vi "App - analyze RUS V6.vi"() -> ()   [LabVIEW 2015] (continued)
"z(0)"=-0.2711634458020681+0.39008831058364485i, "radius"=0.46500524213102634}}, "timestamp(min)"=628.25, "timestamp"=timestamp(3493765516 s since 1904-01-01), "Magn Field(T)"=0.0}, {"temperature"=96.968, "lorentzian"={"Amplitude"=0.00037146242302691187, "omega(0)"=668.0649075247303, "Gamma"=0.06217233966341157, "phase"=3.691468660230438, "Q"=10745.37183483038, "Norm  Ampl"=0.029107990080270388, "z (inf)"=0.2326634260645355-0.3951672463399738i, "4corners"={"z (-pi/2)"=-0.4111672463399738-0.2406634260645355i, "z(inf)"=0.2326634260645355-0.3951672463399738i, "z (pi/2)"=0.3871672463399738+0.2486634260645355i, "z center"=-0.01200000000000001+0.0040000000000000036i, "z(0)"=-0.2566634260645355+0.4031672463399738i, "radius"=0.4681823176971486}}, "timestamp(min)"=629.5666666701436, "timestamp"=timestamp(3493765595 s since 1904-01-01), "Magn Field(T)"=0.0}, {"temperature"=96.812, "lorentzian"={"Amplitude"=0.00038447207921998627, "omega(0)"=668.0660057593828, "Gamma"=0.06696620336364374, "phase"=3.806955565337118, "Q"=9976.166666215378, "Norm  Ampl"=0.030872979781580823, "z (inf)"=0.2726102759872714-0.350683705269581i, "4corners"={"z (-pi/2)"=-0.374683705269581-0.2726102759872714i, "z(inf)"=0.2726102759872714-0.350683705269581i, "z (pi/2)"=0.350683705269581+0.2966102759872714i, "z center"=-0.01200000000000001+0.01200000000000001i, "z(0)"=-0.2966102759872714+0.374683705269581i, "radius"=0.4610232957949339}}, "timestamp(min)"=630.8999999985099, "timestamp"=timestamp(3493765675 s since 1904-01-01), "Magn Field(T)"=0.0}, {"temperature"=96.655, "lorentzian"={"Amplitude"=0.000361199895859237, "omega(0)"=668.0603228410023, "Gamma"=0.0629920810816999, "phase"=3.775356755255857, "Q"=10605.465184973596, "Norm  Ampl"=0.029419314400986003, "z (inf)"=0.25656794858229404-0.372336300708436i, "4corners"={"z (-pi/2)"=-0.396336300708436-0.27256794858229405i, "z(inf)"=0.25656794858229404-0.372336300708436i, "z (pi/2)"=0.35633630070843597+0.28056794858229406i, "z center"=-0.020000000000000018+0.0040000000000000036i, "z(0)"=-0.29656794858229407+0.380336300708436i, "radius"=0.46703194902910955}}, "timestamp(min)"=632.2166666686535, "timestamp"=timestamp(3493765754 s since 1904-01-01), "Magn Field(T)"=0.0}, {"temperature"=96.507, "lorentzian"={"Amplitude"=0.00035745009367951465, "omega(0)"=668.0526848700105, "Gamma"=0.06285914936442166, "phase"=3.782468820239237, "Q"=10627.771639050034, "Norm  Ampl"=0.028980262367324632, "z (inf)"=0.2556518430633841-0.3655527717167506i, "4corners"={"z (-pi/2)"=-0.3895527717167506-0.27165184306338414i, "z(inf)"=0.2556518430633841-0.3655527717167506i, "z (pi/2)"=0.3495527717167506+0.27965184306338414i, "z center"=-0.020000000000000018+0.0040000000000000036i, "z(0)"=-0.29565184306338416+0.3735527717167506i, "radius"=0.4610349115498449}}, "timestamp(min)"=633.5500000044703, "timestamp"=timestamp(3493765834 s since 1904-01-01), "Magn Field(T)"=0.0}, {"temperature"=96.351, "lorentzian"={"Amplitude"=0.0003691797242721114, "omega(0)"=668.0459870419369, "Gamma"=0.06408388530782533, "phase"=3.8227658205621733, "Q"=10424.555000574557, "Norm  Ampl"=0.029587224824382054, "z (inf)"=0.2627317152722984-0.35466079325625405i, "4corners"={"z (-pi/2)"=-0.3866607932562541-0.2867317152722984i, "z(inf)"=0.2627317152722984-0.35466079325625405i, "z (pi/2)"=0.330660793256254+0.2947317152722984i, "z center"=-0.028000000000000025+0.0040000000000000036i, "z(0)"=-0.31873171527229843+0.36266079325625405i, "radius"=0.4616952402661069}}, "timestamp(min)"=634.8666666671634, "timestamp"=timestamp(3493765913 s since 1904-01-01), "Magn Field(T)"=0.0}, {"temperature"=96.204, "lorentzian"={"Amplitude"=0.00038180833108307917, "omega(0)"=668.0382438056512, "Gamma"=0.0652530874331081, "phase"=3.8620996852149454, "Q"=10237.649589997822, "Norm  Ampl"=0.02969485182794312, "z (inf)"=0.27224091953885815-0.33797353554027637i, "4corners"={"z (-pi/2)"=-0.3699735355402764-0.29624091953885817i, "z(inf)"=0.27224091953885815-0.33797353554027637i, "z (pi/2)"=0.31397353554027635+0.3042409195388582i, "z center"=-0.028000000000000025+0.0040000000000000036i, "z(0)"=-0.3282409195388582+0.3459735355402764i, "radius"=0.45507198197148524}}, "timestamp(min)"=636.183333337307, "timestamp"=timestamp(3493765992 s since 1904-01-01), "Magn Field(T)"=0.0}, {"temperature"=96.051, "lorentzian"={"Amplitude"=0.0003882934961133009, "omega(0)"=668.0317727144501, "Gamma"=0.06568797813583101, "phase"=3.9352495822111924, "Q"=10169.772181647602, "Norm  Ampl"=0.02993123400136465, "z (inf)"=0.2888486047387337-0.31552673906111356i, "4corners"={"z (-pi/2)"=-0.35552673906111354-0.32084860473873367i, "z(inf)"=0.2888486047387337-0.31552673906111356i, "z (pi/2)"=0.2835267390611136+0.3288486047387337i, "z center"=-0.035999999999999976+0.0040000000000000036i, "z(0)"=-0.36084860473873365+0.32352673906111357i, "radius"=0.4556577147110876}}, "timestamp(min)"=637.5166666656733, "timestamp"=timestamp(3493766072 s since 1904-01-01), "Magn Field(T)"=0.0}, {"temperature"=95.897, "lorentzian"={"Amplitude"=0.0003815839774204844, "omega(0)"=668.0229320244955, "Gamma"=0.06445033392425954, "phase"=3.977002601298967, "Q"=10364.925848321278, "Norm  Ampl"=0.029097485771713064, "z (inf)"=0.29079840497182946-0.2988803378584398i, "4corners"={"z (-pi/2)"=-0.3468803378584398-0.33079840497182944i, "z(inf)"=0.29079840497182946-0.2988803378584398i, "z (pi/2)"=0.25888033785843984+0.33879840497182945i, "z center"=-0.043999999999999984+0.0040000000000000036i, "z(0)"=-0.3787984049718294+0.3068803378584398i, "radius"=0.45147145096110314}}, "timestamp(min)"=638.8333333358169, "timestamp"=timestamp(3493766151 s since 1904-01-01), "Magn Field(T)"=0.0}, {"temperature"=95.75, "lorentzian"={"Amplitude"=0.0004135836601823012, "omega(0)"=668.0104558389754, "Gamma"=0.06731735153927441, "phase"=3.9838630372883417, "Q"=9923.302693351558, "Norm  Ampl"=0.030634815829311563, "z (inf)"=0.3035613371868464-0.29897918169328014i, "4corners"={"z (-pi/2)"=-0.3389791816932801-0.3355613371868464i, "z(inf)"=0.3035613371868464-0.29897918169328014i, "z (pi/2)"=0.26697918169328017+0.3435613371868464i, "z center"=-0.035999999999999976+0.0040000000000000036i, "z(0)"=-0.37556133718684637+0.30697918169328015i, "radius"=0.45508052721650133}}, "timestamp(min)"=640.1499999985099, "timestamp"=timestamp(3493766230 s since 1904-01-01), "Magn Field(T)"=0.0}, {"temperature"=95.599, "lorentzian"={"Amplitude"=0.00042216802189360146, "omega(0)"=668.0013835956787, "Gamma"=0.06780134474946373, "phase"=3.9776981169897643, "Q"=9852.332369867372, "Norm  Ampl"=0.0307062205288882, "z (inf)"=0.30005798229377045-0.30759507485352017i, "4corners"={"z (-pi/2)"=-0.33959507485352014-0.34005798229377043i, "z(inf)"=0.30005798229377045-0.30759507485352017i, "z (pi/2)"=0.2675950748535202+0.3320579822937704i, "z center"=-0.035999999999999976-0.0040000000000000036i, "z(0)"=-0.3720579822937704+0.29959507485352016i, "radius"=0.4528851255436357}}, "timestamp(min)"=641.4833333343267, "timestamp"=timestamp(3493766310 s since 1904-01-01), "Magn Field(T)"=0.0}, {"temperature"=95.455, "lorentzian"={"Amplitude"=0.0004523874054454233, "omega(0)"=667.9844280868045, "Gamma"=0.06782073622219846, "phase"=3.948222002818395, "Q"=9849.265361825519, "Norm  Ampl"=0.031118440336053946, "z (inf)"=0.3032591325695712-0.32148348753188644i, "4corners"={"z (-pi/2)"=-0.34548348753188646-0.33525913256957124i, "z(inf)"=0.3032591325695712-0.32148348753188644i, "z (pi/2)"=0.2894834875318864+0.32725913256957123i, "z center"=-0.028000000000000025-0.0040000000000000036i, "z(0)"=-0.35925913256957126+0.31348348753188643i, "radius"=0.45883371472261525}}, "timestamp(min)"=642.8000000044703, "timestamp"=timestamp(3493766389 s since 1904-01-01), "Magn Field(T)"=0.0}, {"temperature"=95.306, "lorentzian"={"Amplitude"=0.0004854419287925806, "omega(0)"=667.9730328624377, "Gamma"=0.07037414769947414, "phase"=3.891621301723143, "Q"=9491.738865740166, "Norm  Ampl"=0.032723058122378475, "z (inf)"=0.29696285365839886-0.3442166726157581i, "4corners"={"z (-pi/2)"=-0.3602166726157581-0.3209628536583989i, "z(inf)"=0.29696285365839886-0.3442166726157581i, "z (pi/2)"=0.3202166726157581+0.3129628536583989i, "z center"=-0.020000000000000018-0.0040000000000000036i, "z(0)"=-0.3369628536583989+0.3362166726157581i, "radius"=0.4649869190902186}}, "timestamp(min)"=644.1166666671634, "timestamp"=timestamp(3493766468 s since 1904-01-01), "Magn Field(T)"=0.0}, {"temperature"=95.156, "lorentzian"={"Amplitude"=0.0004910318217417332, "omega(0)"=667.9597690228534, "Gamma"=0.07026492453818647, "phase"=3.8418803163628708, "Q"=9506.304509867383, "Norm  Ampl"=0.03265446304858576, "z (inf)"=0.27949176570968204-0.3593616350093592i, "4corners"={"z (-pi/2)"=-0.3753616350093592-0.30349176570968206i, "z(inf)"=0.27949176570968204-0.3593616350093592i, "z (pi/2)"=0.33536163500935917+0.29549176570968205i, "z center"=-0.020000000000000018-0.0040000000000000036i, "z(0)"=-0.3194917657096821+0.3513616350093592i, "radius"=0.46473348207809184}}, "timestamp(min)"=645.4500000029802, "timestamp"=timestamp(3493766548 s since 1904-01-01), "Magn Field(T)"=0.0}, {"temperature"=95.012, "lorentzian"={"Amplitude"=0.0004787690427261217, "omega(0)"=667.9520044016398, "Gamma"=0.06706732978723035, "phase"=3.8089981908201227, "Q"=9959.424454808372, "Norm  Ampl"=0.031129732965038723, "z (inf)"=0.27528976862458415-0.36056246197020664i, "4corners"={"z (-pi/2)"=-0.37656246197020665-0.28328976862458416i, "z(inf)"=0.27528976862458415-0.36056246197020664i, "z (pi/2)"=0.35256246197020663+0.29128976862458417i, "z center"=-0.01200000000000001+0.0040000000000000036i, "z(0)"=-0.2992897686245842+0.36856246197020665i, "radius"=0.46415643896658965}}, "timestamp(min)"=646.7666666656733, "timestamp"=timestamp(3493766627 s since 1904-01-01), "Magn Field(T)"=0.0}, {"temperature"=94.866, "lorentzian"={"Amplitude"=0.0004761292193022266, "omega(0)"=667.9421204350114, "Gamma"=0.06630831442400692, "phase"=3.797924871572925, "Q"=10073.278535838983, "Norm  Ampl"=0.030739202330990468, "z (inf)"=0.270883513585858-0.363264549434754i, "4corners"={"z (-pi/2)"=-0.379264549434754-0.278883513585858i, "z(inf)"=0.270883513585858-0.363264549434754i, "z (pi/2)"=0.355264549434754+0.286883513585858i, "z center"=-0.01200000000000001+0.0040000000000000036i, "z(0)"=-0.294883513585858+0.371264549434754i, "radius"=0.4635799084626006}}, "timestamp(min)"=648.1000000014901, "timestamp"=timestamp(3493766707 s since 1904-01-01), "Magn Field(T)"=0.0}, {"temperature"=94.718, "lorentzian"={"Amplitude"=0.00047853053416581755, "omega(0)"=667.9314512587483, "Gamma"=0.06647786623615008, "phase"=3.7908834379562117, "Q"=10047.426144606505, "Norm  Ampl"=0.03076620958437617, "z (inf)"=0.2678212054341876-0.36462915903255366i, "4corners"={"z (-pi/2)"=-0.3806291590325537-0.2758212054341876i, "z(inf)"=0.2678212054341876-0.36462915903255366i, "z (pi/2)"=0.35662915903255366+0.2838212054341876i, "z center"=-0.01200000000000001+0.0040000000000000036i, "z(0)"=-0.2918212054341876+0.37262915903255367i, "radius"=0.46280380713612285}}, "timestamp(min)"=649.4166666641831, "timestamp"=timestamp(3493766786 s since 1904-01-01), "Magn Field(T)"=0.0}, {"temperature"=94.578, "lorentzian"={"Amplitude"=0.00047146401355324603, "omega(0)"=667.9245739426502, "Gamma"=0.06593817695384066, "phase"=3.8213286752443887, "Q"=10129.557788809114, "Norm  Ampl"=0.030202816047765486, "z (inf)"=0.2759230326145807-0.3522412452433142i, "4corners"={"z (-pi/2)"=-0.3682412452433142-0.2839230326145807i, "z(inf)"=0.2759230326145807-0.3522412452433142i, "z (pi/2)"=0.3442412452433142+0.2919230326145807i, "z center"=-0.01200000000000001+0.0040000000000000036i, "z(0)"=-0.2999230326145807+0.3602412452433142i, "radius"=0.45804748391677036}}, "timestamp(min)"=650.7333333343267, "timestamp"=timestamp(3493766865 s since 1904-01-01), "Magn Field(T)"=0.0}, {"temperature"=94.43, "lorentzian"={"Amplitude"=0.00047892263818113853, "omega(0)"=667.915672183135, "Gamma"=0.06684496153277945, "phase"=3.8401916398474936, "Q"=9992.012215544508, "Norm  Ampl"=0.0307040161855886, "z (inf)"=0.2834171775596786-0.3557305635687633i, "4corners"={"z (-pi/2)"=-0.3637305635687633-0.2994171775596786i, "z(inf)"=0.2834171775596786-0.3557305635687633i, "z (pi/2)"=0.3397305635687633+0.2914171775596786i, "z center"=-0.01200000000000001-0.0040000000000000036i, "z(0)"=-0.3074171775596786+0.3477305635687633i, "radius"=0.45933179526974455}}, "timestamp(min)"=652.0666666701436, "timestamp"=timestamp(3493766945 s since 1904-01-01), "Magn Field(T)"=0.0}, {"temperature"=94.292, "lorentzian"={"Amplitude"=0.0004657252078627852, "omega(0)"=667.9042185316268, "Gamma"=0.06477161400596823, "phase"=3.8153255665284904, "Q"=10311.680954408273, "Norm  Ampl"=0.029982133107207858, "z (inf)"=0.2768005918537779-0.3577476748367419i, "4corners"={"z (-pi/2)"=-0.3737476748367419-0.28480059185377793i, "z(inf)"=0.2768005918537779-0.3577476748367419i, "z (pi/2)"=0.3497476748367419+0.29280059185377794i, "z center"=-0.01200000000000001+0.0040000000000000036i, "z(0)"=-0.30080059185377794+0.3657476748367419i, "radius"=0.46289001080697517}}, "timestamp(min)"=653.3833333328366, "timestamp"=timestamp(3493767024 s since 1904-01-01), "Magn Field(T)"=0.0}, {"temperature"=94.146, "lorentzian"={"Amplitude"=0.00047004334807755914, "omega(0)"=667.8931568087993, "Gamma"=0.06620722920307591, "phase"=3.794159084218575, "Q"=10087.918870010191, "Norm  Ampl"=0.030640583697349073, "z (inf)"=0.26902377025013874-0.3637060990321072i, "4corners"={"z (-pi/2)"=-0.3797060990321072-0.27702377025013875i, "z(inf)"=0.26902377025013874-0.3637060990321072i, "z (pi/2)"=0.3557060990321072+0.28502377025013875i, "z center"=-0.01200000000000001+0.0040000000000000036i, "z(0)"=-0.29302377025013876+0.3717060990321072i, "radius"=0.4627981576357155}}, "timestamp(min)"=654.7000000029802, "timestamp"=timestamp(3493767103 s since 1904-01-01), "Magn Field(T)"=0.0}, {"temperature"=94.003, "lorentzian"={"Amplitude"=0.00047665410550718444, "omega(0)"=667.8785430669695, "Gamma"=0.06600452228276824, "phase"=3.7493809753851632, "Q"=10118.678538505721, "Norm  Ampl"=0.030401685578484956, "z (inf)"=0.25102715548226634-0.3741125652184201i, "4corners"={"z (-pi/2)"=-0.39011256521842014-0.25902715548226635i, "z(inf)"=0.25102715548226634-0.3741125652184201i, "z (pi/2)"=0.3661125652184201+0.26702715548226635i, "z center"=-0.01200000000000001+0.0040000000000000036i, "z(0)"=-0.27502715548226636+0.38211256521842013i, "radius"=0.4606000396191324}}, "timestamp(min)"=656.0333333313465, "timestamp"=timestamp(3493767183 s since 1904-01-01), "Magn Field(T)"=0.0}, {"temperature"=93.867, "lorentzian"={"Amplitude"=0.00048650304629364036, "omega(0)"=667.867203293899, "Gamma"=0.06682589428323253, "phase"=3.7348237629828676, "Q"=9994.137908027598, "Norm  Ampl"=0.03108362649647347, "z (inf)"=0.24803517339436904-0.38166842033020015i, "4corners"={"z (-pi/2)"=-0.39766842033020017-0.25603517339436904i, "z(inf)"=0.24803517339436904-0.38166842033020015i, "z (pi/2)"=0.37366842033020015+0.26403517339436905i, "z center"=-0.01200000000000001+0.0040000000000000036i, "z(0)"=-0.27203517339436906+0.38966842033020016i, "radius"=0.46514344222210796}}, "timestamp(min)"=657.3500000014901, "timestamp"=timestamp(3493767262 s since 1904-01-01), "Magn Field(T)"=0.0}, {"temperature"=93.722, "lorentzian"={"Amplitude"=0.0004956688777062957, "omega(0)"=667.8547807071961, "Gamma"=0.0674977463368087, "phase"=3.7437605166589782, "Q"=9894.47525217584, "Norm  Ampl"=0.03128536274271491, "z (inf)"=0.2505417919292505-0.3859767244686182i, "4corners"={"z (-pi/2)"=-0.3939767244686182-0.26654179192925054i, "z(inf)"=0.2505417919292505-0.3859767244686182i, "z (pi/2)"=0.3699767244686182+0.25854179192925053i, "z center"=-0.01200000000000001-0.0040000000000000036i, "z(0)"=-0.27454179192925054+0.3779767244686182i, "radius"=0.46350233067935753}}, "timestamp(min)"=658.683333337307, "timestamp"=timestamp(3493767342 s since 1904-01-01), "Magn Field(T)"=0.0}, {"temperature"=93.585, "lorentzian"={"Amplitude"=0.000482384363144179, "omega(0)"=667.8418460648647, "Gamma"=0.06604388460816402, "phase"=3.731195401069006, "Q"=10112.092134300492, "Norm  Ampl"=0.030626323452688318, "z (inf)"=0.24584645857021942-0.38143197531309236i, "4corners"={"z (-pi/2)"=-0.3974319753130924-0.2538464585702194i, "z(inf)"=0.24584645857021942-0.38143197531309236i, "z (pi/2)"=0.37343197531309236+0.26184645857021943i, "z center"=-0.01200000000000001+0.0040000000000000036i, "z(0)"=-0.26984645857021944+0.38943197531309237i, "radius"=0.4637268633484113}}, "timestamp(min)"=660.0, "timestamp"=timestamp(3493767421 s since 1904-01-01), "Magn Field(T)"=0.0}, {"temperature"=93.444, "lorentzian"={"Amplitude"=0.00048781220349119976, "omega(0)"=667.8284078259741, "Gamma"=0.06779248490994184, "phase"=3.7207259148041842, "Q"=9851.068429091265, "Norm  Ampl"=0.031501770847735304, "z (inf)"=0.24231844551293596-0.38490753149851276i, "4corners"={"z (-pi/2)"=-0.40090753149851277-0.25031844551293597i, "z(inf)"=0.24231844551293596-0.38490753149851276i, "z (pi/2)"=0.37690753149851275+0.258318445512936i, "z center"=-0.01200000000000001+0.0040000000000000036i, "z(0)"=-0.266318445512936+0.39290753149851276i, "radius"=0.46467939461997115}}, "timestamp(min)"=661.3166666701436, "timestamp"=timestamp(3493767500 s since 1904-01-01), "Magn Field(T)"=0.0}, {"temperature"=93.303, "lorentzian"={"Amplitude"=0.0004977863242643817, "omega(0)"=667.8174456972619, "Gamma"=0.06925915720810301, "phase"=3.733369961748711, "Q"=9642.298182905555, "Norm  Ampl"=0.03210673818426036, "z (inf)"=0.2465986694380145-0.3887434164619287i, "4corners"={"z (-pi/2)"=-0.39674341646192873-0.2625986694380145i, "z(inf)"=0.2465986694380145-0.3887434164619287i, "z (pi/2)"=0.3727434164619287+0.2545986694380145i, "z center"=-0.01200000000000001-0.0040000000000000036i, "z(0)"=-0.2705986694380145+0.3807434164619287i, "radius"=0.463573908180679}}, "timestamp(min)"=662.6499999985099, "timestamp"=timestamp(3493767580 s since 1904-01-01), "Magn Field(T)"=0.0}, {"temperature"=93.168, "lorentzian"={"Amplitude"=0.00048225409501391443, "omega(0)"=667.8098934060879, "Gamma"=0.06771518067251926, "phase"=3.7456795533249925, "Q"=9862.04107814046, "Norm  Ampl"=0.031358841542932885, "z (inf)"=0.2510453154387986-0.3771403549090192i, "4corners"={"z (-pi/2)"=-0.3931403549090192-0.2590453154387986i, "z(inf)"=0.2510453154387986-0.3771403549090192i, "z (pi/2)"=0.3691403549090192+0.2670453154387986i, "z center"=-0.01200000000000001+0.0040000000000000036i, "z(0)"=-0.2750453154387986+0.3851403549090192i, "radius"=0.46309913421908944}}, "timestamp(min)"=663.9666666686535, "timestamp"=timestamp(3493767659 s since 1904-01-01), "Magn Field(T)"=0.0}, {"temperature"=93.028, "lorentzian"={"Amplitude"=0.0004824745179479892, "omega(0)"=667.7999931838958, "Gamma"=0.06758256658053667, "phase"=3.763405165125436, "Q"=9881.246406765169, "Norm  Ampl"=0.031281978812503275, "z (inf)"=0.25762642400328667-0.38023227467776743i, "4corners"={"z (-pi/2)"=-0.38823227467776744-0.2736264240032867i, "z(inf)"=0.25762642400328667-0.38023227467776743i, "z (pi/2)"=0.3642322746777674+0.2656264240032867i, "z center"=-0.01200000000000001-0.0040000000000000036i, "z(0)"=-0.2816264240032867+0.3722322746777674i, "radius"=0.4628705359277119}}, "timestamp(min)"=665.2833333313465, "timestamp"=timestamp(3493767738 s since 1904-01-01), "Magn Field(T)"=0.0}, {"temperature"=92.895, "lorentzian"={"Amplitude"=0.00046952632702334146, "omega(0)"=667.7879029943412, "Gamma"=0.0659901281238434, "phase"=3.723190998312637, "Q"=10119.512144924258, "Norm  Ampl"=0.030488656955698742, "z (inf)"=0.24181454637365946-0.3820559902589959i, "4corners"={"z (-pi/2)"=-0.3980559902589959-0.24981454637365946i, "z(inf)"=0.24181454637365946-0.3820559902589959i, "z (pi/2)"=0.3740559902589959+0.25781454637365947i, "z center"=-0.01200000000000001+0.0040000000000000036i, "z(0)"=-0.2658145463736595+0.3900559902589959i, "radius"=0.46201845370690603}}, "timestamp(min)"=666.6166666671634, "timestamp"=timestamp(3493767818 s since 1904-01-01), "Magn Field(T)"=0.0}, {"temperature"=92.755, "lorentzian"={"Amplitude"=0.0004533781628719222, "omega(0)"=667.7767811952523, "Gamma"=0.06357707675527592, "phase"=3.7161636244174314, "Q"=10503.420655304619, "Norm  Ampl"=0.029386934028224773, "z (inf)"=0.23120776305430374-0.38400373351334605i, "4corners"={"z (-pi/2)"=-0.40800373351334607-0.24720776305430375i, "z(inf)"=0.23120776305430374-0.38400373351334605i, "z (pi/2)"=0.36800373351334603+0.25520776305430376i, "z center"=-0.020000000000000018+0.0040000000000000036i, "z(0)"=-0.2712077630543038+0.39200373351334605i, "radius"=0.4622253102536066}}, "timestamp(min)"=667.933333337307, "timestamp"=timestamp(3493767897 s since 1904-01-01), "Magn Field(T)"=0.0}, {"temperature"=92.618, "lorentzian"={"Amplitude"=0.0004725360269472116, "omega(0)"=667.766686685923, "Gamma"=0.06603299924648035, "phase"=3.718541594649695, "Q"=10112.620876016259, "Norm  Ampl"=0.03057472850998967, "z (inf)"=0.2405642593646345-0.384072966292819i, "4corners"={"z (-pi/2)"=-0.400072966292819-0.2485642593646345i, "z(inf)"=0.2405642593646345-0.384072966292819i, "z (pi/2)"=0.376072966292819+0.2565642593646345i, "z center"=-0.01200000000000001+0.0040000000000000036i, "z(0)"=-0.2645642593646345+0.392072966292819i, "radius"=0.4630219565805857}}, "timestamp(min)"=669.2666666656733, "timestamp"=timestamp(3493767977 s since 1904-01-01), "Magn Field(T)"=0.0}, {"temperature"=92.485, "lorentzian"={"Amplitude"=0.0004628266939696805, "omega(0)"=667.7537699797824, "Gamma"=0.06509770931054754, "phase"=3.7185205526120066, "Q"=10257.71531828062, "Norm  Ampl"=0.030151235786846406, "z (inf)"=0.2326362554983411-0.3842014578439372i, "4corners"={"z (-pi/2)"=-0.40820145784393724-0.24863625549834112i, "z(inf)"=0.2326362554983411-0.3842014578439372i, "z (pi/2)"=0.3682014578439372+0.2566362554983411i, "z center"=-0.020000000000000018+0.0040000000000000036i, "z(0)"=-0.27263625549834114+0.39220145784393723i, "radius"=0.4631689210907628}}, "timestamp(min)"=670.5833333358169, "timestamp"=timestamp(3493768056 s since 1904-01-01), "Magn Field(T)"=0.0}, {"temperature"=92.348, "lorentzian"={"Amplitude"=0.0004709340282676857, "omega(0)"=667.7441411520185, "Gamma"=0.06634297124541383, "phase"=3.7335153124062965, "Q"=10065.032189799285, "Norm  Ampl"=0.030723334211136075, "z (inf)"=0.23838936327255184-0.3803113449909337i, "4corners"={"z (-pi/2)"=-0.40431134499093374-0.25438936327255185i, "z(inf)"=0.23838936327255184-0.3803113449909337i, "z (pi/2)"=0.3643113449909337+0.26238936327255186i, "z center"=-0.020000000000000018+0.0040000000000000036i, "z(0)"=-0.27838936327255187+0.3883113449909337i, "radius"=0.46309855640148057}}, "timestamp(min)"=671.8999999985099, "timestamp"=timestamp(3493768135 s since 1904-01-01), "Magn Field(T)"=0.0}, {"temperature"=92.218, "lorentzian"={"Amplitude"=0.0004646839205690204, "omega(0)"=667.7346507175026, "Gamma"=0.0656240651590833, "phase"=3.75255081841295, "Q"=10175.149148392535, "Norm  Ampl"=0.030385059677175152, "z (inf)"=0.24561090162017518-0.3752566651128105i, "4corners"={"z (-pi/2)"=-0.3992566651128105-0.2616109016201752i, "z(inf)"=0.24561090162017518-0.3752566651128105i, "z (pi/2)"=0.35925666511281046+0.2696109016201752i, "z center"=-0.020000000000000018+0.0040000000000000036i, "z(0)"=-0.2856109016201752+0.3832566651128105i, "radius"=0.46301702894383145}}, "timestamp(min)"=673.2333333343267, "timestamp"=timestamp(3493768215 s since 1904-01-01), "Magn Field(T)"=0.0}, {"temperature"=92.082, "lorentzian"={"Amplitude"=0.0004749862394250107, "omega(0)"=667.7218411788447, "Gamma"=0.06705767219373826, "phase"=3.7603842163008987, "Q"=9957.426485812244, "Norm  Ampl"=0.03103865948557628, "z (inf)"=0.24848549273528175-0.37304069686884916i, "4corners"={"z (-pi/2)"=-0.3970406968688492-0.26448549273528177i, "z(inf)"=0.24848549273528175-0.37304069686884916i, "z (pi/2)"=0.35704069686884915+0.2724854927352818i, "z center"=-0.020000000000000018+0.0040000000000000036i, "z(0)"=-0.2884854927352818+0.38104069686884917i, "radius"=0.4628651498057014}}, "timestamp(min)"=674.5500000044703, "timestamp"=timestamp(3493768294 s since 1904-01-01), "Magn Field(T)"=0.0}, {"temperature"=91.948, "lorentzian"={"Amplitude"=0.00048240630679528417, "omega(0)"=667.7090832290504, "Gamma"=0.06807373016118351, "phase"=3.761077209038164, "Q"=9808.61606449453, "Norm  Ampl"=0.031227719593183583, "z (inf)"=0.23834797737965352-0.36949087855823637i, "4corners"={"z (-pi/2)"=-0.4014908785582364-0.26234797737965354i, "z(inf)"=0.23834797737965352-0.36949087855823637i, "z (pi/2)"=0.34549087855823635+0.27034797737965355i, "z center"=-0.028000000000000025+0.0040000000000000036i, "z(0)"=-0.29434797737965357+0.3774908785582364i, "radius"=0.4587337805529866}}, "timestamp(min)"=675.8666666671634, "timestamp"=timestamp(3493768373 s since 1904-01-01), "Magn Field(T)"=0.0}, {"temperature"=91.818, "lorentzian"={"Amplitude"=0.00046187913692467586, "omega(0)"=667.6987650095127, "Gamma"=0.06501069688502076, "phase"=3.7818049219720504, "Q"=10270.598486129418, "Norm  Ampl"=0.029800728728416378, "z (inf)"=0.24583082565039227-0.3636204223463083i, "4corners"={"z (-pi/2)"=-0.39562042234630834-0.2698308256503923i, "z(inf)"=0.24583082565039227-0.3636204223463083i, "z (pi/2)"=0.3396204223463083+0.2778308256503923i, "z center"=-0.028000000000000025+0.0040000000000000036i, "z(0)"=-0.3018308256503923+0.3716204223463083i, "radius"=0.45839731238572246}}, "timestamp(min)"=677.2000000029802, "timestamp"=timestamp(3493768453 s since 1904-01-01), "Magn Field(T)"=0.0}, {"temperature"=91.685, "lorentzian"={"Amplitude"=0.00048772981058133426, "omega(0)"=667.6847550615028, "Gamma"=0.06909515397897131, "phase"=3.8213110627573736, "Q"=9663.264593993214, "Norm  Ampl"=0.03163038100550472, "z (inf)"=0.25174863771982026-0.35203829662944414i, "4corners"={"z (-pi/2)"=-0.3920382966294441-0.28374863771982023i, "z(inf)"=0.25174863771982026-0.35203829662944414i, "z (pi/2)"=0.32003829662944416+0.29174863771982024i, "z center"=-0.035999999999999976+0.0040000000000000036i, "z(0)"=-0.3237486377198202+0.36003829662944414i, "radius"=0.45778002050811306}}, "timestamp(min)"=678.5166666656733, "timestamp"=timestamp(3493768532 s since 1904-01-01), "Magn Field(T)"=0.0}, {"temperature"=91.557, "lorentzian"={"Amplitude"=0.0004936970308438804, "omega(0)"=667.6716677581467, "Gamma"=0.06917469758289295, "phase"=3.7984123962847027, "Q"=9651.96366717855, "Norm  Ampl"=0.03174648182411007, "z (inf)"=0.2522245068977959-0.35944573170689686i, "4corners"={"z (-pi/2)"=-0.3914457317068969-0.27622450689779593i, "z(inf)"=0.2522245068977959-0.35944573170689686i, "z (pi/2)"=0.33544573170689684+0.28422450689779594i, "z center"=-0.028000000000000025+0.0040000000000000036i, "z(0)"=-0.30822450689779596+0.36744573170689687i, "radius"=0.45893199295982245}}, "timestamp(min)"=679.8500000014901, "timestamp"=timestamp(3493768612 s since 1904-01-01), "Magn Field(T)"=0.0}, {"temperature"=91.423, "lorentzian"={"Amplitude"=0.0005094399076372343, "omega(0)"=667.6622092104991, "Gamma"=0.07106029145812462, "phase"=3.881324924167042, "Q"=9395.71447724709, "Norm  Ampl"=0.03277559689637478, "z (inf)"=0.2829149636577557-0.3366918731694022i, "4corners"={"z (-pi/2)"=-0.3686918731694022-0.3069149636577557i, "z(inf)"=0.2829149636577557-0.3366918731694022i, "z (pi/2)"=0.31269187316940217+0.31491496365775573i, "z center"=-0.028000000000000025+0.0040000000000000036i, "z(0)"=-0.33891496365775575+0.3446918731694022i, "radius"=0.4612364546195147}}, "timestamp(min)"=681.1666666641831, "timestamp"=timestamp(3493768691 s since 1904-01-01), "Magn Field(T)"=0.0}, {"temperature"=91.291, "lorentzian"={"Amplitude"=0.0005088040446388636, "omega(0)"=667.6494194591486, "Gamma"=0.07122298109703128, "phase"=3.860166057202675, "Q"=9374.072935104616, "Norm  Ampl"=0.03258903067532576, "z (inf)"=0.27321925003049036-0.34042886777923675i, "4corners"={"z (-pi/2)"=-0.3724288677792368-0.2972192500304904i, "z(inf)"=0.27321925003049036-0.34042886777923675i, "z (pi/2)"=0.31642886777923673+0.3052192500304904i, "z center"=-0.028000000000000025+0.0040000000000000036i, "z(0)"=-0.3292192500304904+0.34842886777923676i, "radius"=0.4575634180620409}}, "timestamp(min)"=682.4833333343267, "timestamp"=timestamp(3493768770 s since 1904-01-01), "Magn Field(T)"=0.0}, {"temperature"=91.167, "lorentzian"={"Amplitude"=0.000510744332757808, "omega(0)"=667.6370796373111, "Gamma"=0.0716029354059644, "phase"=3.865224682997533, "Q"=9324.157953190535, "Norm  Ampl"=0.03278392731323275, "z (inf)"=0.27515231362484527-0.34712095541253063i, "4corners"={"z (-pi/2)"=-0.37112095541253065-0.3071523136248453i, "z(inf)"=0.27515231362484527-0.34712095541253063i, "z (pi/2)"=0.3151209554125306+0.2991523136248453i, "z center"=-0.028000000000000025-0.0040000000000000036i, "z(0)"=-0.3311523136248453+0.3391209554125306i, "radius"=0.45785730888487997}}, "timestamp(min)"=683.8166666701436, "timestamp"=timestamp(3493768850 s since 1904-01-01), "Magn Field(T)"=0.0}, {"temperature"=91.035, "lorentzian"={"Amplitude"=0.0005141802984750622, "omega(0)"=667.6271523663532, "Gamma"=0.0719675199748464, "phase"=3.826833710973994, "Q"=9276.784202091412, "Norm  Ampl"=0.032806058987522896, "z (inf)"=0.2524861359147123-0.3489457864081325i, "4corners"={"z (-pi/2)"=-0.3889457864081325-0.2844861359147123i, "z(inf)"=0.2524861359147123-0.3489457864081325i, "z (pi/2)"=0.31694578640813253+0.2924861359147123i, "z center"=-0.035999999999999976+0.0040000000000000036i, "z(0)"=-0.32448613591471226+0.3569457864081325i, "radius"=0.45584534521946907}}, "timestamp(min)"=685.1333333328366, "timestamp"=timestamp(3493768929 s since 1904-01-01), "Magn Field(T)"=0.0}, {"temperature"=90.91, "lorentzian"={"Amplitude"=0.0005028221303766884, "omega(0)"=667.616063077065, "Gamma"=0.07025360423713384, "phase"=3.8495426280010117, "Q"=9502.943946101263, "Norm  Ampl"=0.03210925964867006, "z (inf)"=0.26120805162066535-0.34321768770733674i, "4corners"={"z (-pi/2)"=-0.3832176877073367-0.2932080516206653i, "z(inf)"=0.26120805162066535-0.34321768770733674i, "z (pi/2)"=0.31121768770733677+0.30120805162066533i, "z center"=-0.035999999999999976+0.0040000000000000036i, "z(0)"=-0.3332080516206653+0.35121768770733675i, "radius"=0.45704786248814433}}, "timestamp(min)"=686.4500000029802, "timestamp"=timestamp(3493769008 s since 1904-01-01), "Magn Field(T)"=0.0}, {"temperature"=90.778, "lorentzian"={"Amplitude"=0.000496497929184537, "omega(0)"=667.5996159742031, "Gamma"=0.06890055492897058, "phase"=3.859639780398612, "Q"=9689.32132204784, "Norm  Ampl"=0.03137956944971089, "z (inf)"=0.26363614673359875-0.33898275837264435i, "4corners"={"z (-pi/2)"=-0.37898275837264433-0.2956361467335987i, "z(inf)"=0.26363614673359875-0.33898275837264435i, "z (pi/2)"=0.3069827583726444+0.30363614673359873i, "z center"=-0.035999999999999976+0.0040000000000000036i, "z(0)"=-0.3356361467335987+0.34698275837264436i, "radius"=0.4554327535106214}}, "timestamp(min)"=687.7833333313465, "timestamp"=timestamp(3493769088 s since 1904-01-01), "Magn Field(T)"=0.0}, {"temperature"=90.65, "lorentzian"={"Amplitude"=0.000499948600021398, "omega(0)"=667.5849862740106, "Gamma"=0.06954975580707387, "phase"=3.849891148655935, "Q"=9598.667580168712, "Norm  Ampl"=0.03138623678832294, "z (inf)"=0.25757515087784166-0.3387316327279606i, "4corners"={"z (-pi/2)"=-0.37873163272796057-0.28957515087784164i, "z(inf)"=0.25757515087784166-0.3387316327279606i, "z (pi/2)"=0.3067316327279606+0.29757515087784164i, "z center"=-0.035999999999999976+0.0040000000000000036i, "z(0)"=-0.3295751508778416+0.3467316327279606i, "radius"=0.4512774548826045}}, "timestamp(min)"=689.1000000014901, "timestamp"=timestamp(3493769167 s since 1904-01-01), "Magn Field(T)"=0.0}, {"temperature"=90.526, "lorentzian"={"Amplitude"=0.0005221121875696492, "omega(0)"=667.5706432660058, "Gamma"=0.0719106912079188, "phase"=3.8795533190442146, "Q"=9283.329530734547, "Norm  Ampl"=0.03259818591965365, "z (inf)"=0.2689814193704261-0.33138143772648987i, "4corners"={"z (-pi/2)"=-0.37138143772648985-0.30098141937042605i, "z(inf)"=0.2689814193704261-0.33138143772648987i, "z (pi/2)"=0.2993814377264899+0.30898141937042606i, "z center"=-0.035999999999999976+0.0040000000000000036i, "z(0)"=-0.34098141937042603+0.3393814377264899i, "radius"=0.4533148739371862}}, "timestamp(min)"=690.4166666641831, "timestamp"=timestamp(3493769246 s since 1904-01-01), "Magn Field(T)"=0.0}, {"temperature"=90.397, "lorentzian"={"Amplitude"=0.0005333126804893269, "omega(0)"=667.555832927336, "Gamma"=0.07307015936595498, "phase"=3.867011857823234, "Q"=9135.82013122535, "Norm  Ampl"=0.03301691741317805, "z (inf)"=0.2637810086163199-0.3340855235035937i, "4corners"={"z (-pi/2)"=-0.3740855235035937-0.2957810086163199i, "z(inf)"=0.2637810086163199-0.3340855235035937i, "z (pi/2)"=0.30208552350359374+0.3037810086163199i, "z center"=-0.035999999999999976+0.0040000000000000036i, "z(0)"=-0.3357810086163199+0.3420855235035937i, "radius"=0.4518522704709107}}, "timestamp(min)"=691.75, "timestamp"=timestamp(3493769326 s since 1904-01-01), "Magn Field(T)"=0.0}, {"temperature"=90.276, "lorentzian"={"Amplitude"=0.0005418855418945078, "omega(0)"=667.5428492141318, "Gamma"=0.07467380998758522, "phase"=3.887607241567496, "Q"=8939.450783683238, "Norm  Ampl"=0.03363448014434847, "z (inf)"=0.2697069491564103-0.32678733838832924i, "4corners"={"z (-pi/2)"=-0.3667873383883292-0.3017069491564103i, "z(inf)"=0.2697069491564103-0.32678733838832924i, "z (pi/2)"=0.29478733838832927+0.3097069491564103i, "z center"=-0.035999999999999976+0.0040000000000000036i, "z(0)"=-0.34170694915641026+0.33478733838832925i, "radius"=0.45041869632660125}}, "timestamp(min)"=693.0666666701436, "timestamp"=timestamp(3493769405 s since 1904-01-01), "Magn Field(T)"=0.0}, {"temperature"=90.146, "lorentzian"={"Amplitude"=0.0005383860372345941, "omega(0)"=667.5298004796668, "Gamma"=0.07451715162242341, "phase"=3.9161664970687338, "Q"=8958.06919542529, "Norm  Ampl"=0.03359771044199378, "z (inf)"=0.27934521178027827-0.3182469832294711i, "4corners"={"z (-pi/2)"=-0.35824698322947107-0.31134521178027824i, "z(inf)"=0.27934521178027827-0.3182469832294711i, "z (pi/2)"=0.2862469832294711+0.31934521178027825i, "z center"=-0.035999999999999976+0.0040000000000000036i, "z(0)"=-0.3513452117802782+0.3262469832294711i, "radius"=0.45087217788775075}}, "timestamp(min)"=694.3999999985099, "timestamp"=timestamp(3493769485 s since 1904-01-01), "Magn Field(T)"=0.0}, {"temperature"=90.022, "lorentzian"={"Amplitude"=0.0005369869284641813, "omega(0)"=667.515440025869, "Gamma"=0.07346468132165142, "phase"=3.9285399901576525, "Q"=9086.208883194866, "Norm  Ampl"=0.03310108006313499, "z (inf)"=0.2830952386772431-0.3221080995718404i, "4corners"={"z (-pi/2)"=-0.35410809957184036-0.3230952386772431i, "z(inf)"=0.2830952386772431-0.3221080995718404i, "z (pi/2)"=0.2821080995718404+0.3150952386772431i, "z center"=-0.035999999999999976-0.0040000000000000036i, "z(0)"=-0.3550952386772431+0.3141080995718404i, "radius"=0.4505713421420571}}, "timestamp(min)"=695.7166666686535, "timestamp"=timestamp(3493769564 s since 1904-01-01), "Magn Field(T)"=0.0}, {"temperature"=89.9, "lorentzian"={"Amplitude"=0.0005373257136341487, "omega(0)"=667.4995586436626, "Gamma"=0.07392447525649636, "phase"=3.952841668349203, "Q"=9029.479835029386, "Norm  Ampl"=0.0332370154898045, "z (inf)"=0.28203205736696485-0.30559684782106095i, "4corners"={"z (-pi/2)"=-0.35359684782106093-0.32203205736696483i, "z(inf)"=0.28203205736696485-0.30559684782106095i, "z (pi/2)"=0.26559684782106097+0.33003205736696484i, "z center"=-0.043999999999999984+0.0040000000000000036i, "z(0)"=-0.3700320573669648+0.31359684782106095i, "radius"=0.4496077297063219}}, "timestamp(min)"=697.0333333313465, "timestamp"=timestamp(3493769643 s since 1904-01-01), "Magn Field(T)"=0.0}, {"temperature"=89.775, "lorentzian"={"Amplitude"=0.0005245742485428037, "omega(0)"=667.4860922618307, "Gamma"=0.07183974762554388, "phase"=3.9569562650148655, "Q"=9291.3201162819, "Norm  Ampl"=0.03235901852579227, "z (inf)"=0.2839041944139377-0.30481879207285606i, "4corners"={"z (-pi/2)"=-0.35281879207285605-0.3239041944139377i, "z(inf)"=0.2839041944139377-0.30481879207285606i, "z (pi/2)"=0.2648187920728561+0.3319041944139377i, "z center"=-0.043999999999999984+0.0040000000000000036i, "z(0)"=-0.3719041944139377+0.31281879207285607i, "radius"=0.4504333547280789}}, "timestamp(min)"=698.3666666671634, "timestamp"=timestamp(3493769723 s since 1904-01-01), "Magn Field(T)"=0.0}, {"temperature"=89.652, "lorentzian"={"Amplitude"=0.000526787378510794, "omega(0)"=667.4736345533211, "Gamma"=0.0723525475330686, "phase"=3.986557210276321, "Q"=9225.295546756712, "Norm  Ampl"=0.03258042651007157, "z (inf)"=0.29280156702488774-0.2948908161645626i, "4corners"={"z (-pi/2)"=-0.3428908161645626-0.3328015670248877i, "z(inf)"=0.29280156702488774-0.2948908161645626i, "z (pi/2)"=0.2548908161645626+0.34080156702488773i, "z center"=-0.043999999999999984+0.0040000000000000036i, "z(0)"=-0.3808015670248877+0.3028908161645626i, "radius"=0.4503010276891874}}, "timestamp(min)"=699.683333337307, "timestamp"=timestamp(3493769802 s since 1904-01-01), "Magn Field(T)"=0.0}, {"temperature"=89.531, "lorentzian"={"Amplitude"=0.0005395240241546807, "omega(0)"=667.4573357267553, "Gamma"=0.07395596056869737, "phase"=3.964431750276373, "Q"=9025.064789832013, "Norm  Ampl"=0.033318481278635834, "z (inf)"=0.28626553214710015-0.3024164205081319i, "4corners"={"z (-pi/2)"=-0.3504164205081319-0.32626553214710013i, "z(inf)"=0.28626553214710015-0.3024164205081319i, "z (pi/2)"=0.2624164205081319+0.33426553214710014i, "z center"=-0.043999999999999984+0.0040000000000000036i, "z(0)"=-0.3742655321471001+0.3104164205081319i, "radius"=0.45051786255533033}}, "timestamp(min)"=701.0, "timestamp"=timestamp(3493769881 s since 1904-01-01), "Magn Field(T)"=0.0}, {"temperature"=89.405, "lorentzian"={"Amplitude"=0.0005332956629755601, "omega(0)"=667.4424028954636, "Gamma"=0.07307309164625458, "phase"=3.9942650823942554, "Q"=9133.901246802849, "Norm  Ampl"=0.03248512410546218, "z (inf)"=0.28276954821470657-0.2885062515458003i, "4corners"={"z (-pi/2)"=-0.3445062515458003-0.33076954821470655i, "z(inf)"=0.28276954821470657-0.2885062515458003i, "z (pi/2)"=0.2405062515458003+0.33876954821470656i, "z center"=-0.05199999999999999+0.0040000000000000036i, "z(0)"=-0.38676954821470655+0.2965062515458003i, "radius"=0.4445565853805944}}, "timestamp(min)"=702.3333333358169, "timestamp"=timestamp(3493769961 s since 1904-01-01), "Magn Field(T)"=0.0}, {"temperature"=89.288, "lorentzian"={"Amplitude"=0.0005440140477486456, "omega(0)"=667.4251980802276, "Gamma"=0.0743822262774763, "phase"=4.064066173569398, "Q"=8972.912367404238, "Norm  Ampl"=0.03297226363889546, "z (inf)"=0.30133864811207084-0.2636756875492752i, "4corners"={"z (-pi/2)"=-0.31967568754927517-0.3493386481120708i, "z(inf)"=0.30133864811207084-0.2636756875492752i, "z (pi/2)"=0.21567568754927519+0.35733864811207083i, "z center"=-0.05199999999999999+0.0040000000000000036i, "z(0)"=-0.4053386481120708+0.2716756875492752i, "radius"=0.443281483884273}}, "timestamp(min)"=703.6499999985099, "timestamp"=timestamp(3493770040 s since 1904-01-01), "Magn Field(T)"=0.0}, {"temperature"=89.165, "lorentzian"={"Amplitude"=0.0005557299049532174, "omega(0)"=667.41000498982, "Gamma"=0.07517572778505581, "phase"=4.091541941986028, "Q"=8877.998586167256, "Norm  Ampl"=0.03331937598483453, "z (inf)"=0.3085088363216765-0.2538317831981052i, "4corners"={"z (-pi/2)"=-0.30983178319810517-0.3565088363216765i, "z(inf)"=0.3085088363216765-0.2538317831981052i, "z (pi/2)"=0.2058317831981052+0.3645088363216765i, "z center"=-0.05199999999999999+0.0040000000000000036i, "z(0)"=-0.4125088363216765+0.2618317831981052i, "radius"=0.44321986586018913}}, "timestamp(min)"=704.9833333343267, "timestamp"=timestamp(3493770120 s since 1904-01-01), "Magn Field(T)"=0.0}, {"temperature"=89.042, "lorentzian"={"Amplitude"=0.0005567343497334853, "omega(0)"=667.3944561053353, "Gamma"=0.07552863492951167, "phase"=4.105063397378044, "Q"=8836.310317645646, "Norm  Ampl"=0.033462211880352005, "z (inf)"=0.31181439331444616-0.2488311548963799i, 
